vi "读取Description.vi"(8 "error in (no error)":errorcluster caption="错误输入（无错误）", 11 "Beverage输入":refnum<class "Beverage.lvclass">) -> (0 "error out":errorcluster caption="错误输出", 2 "Description":string="Unknown Description", 3 "Beverage输出":refnum<class "Beverage.lvclass">)   [LabVIEW 2016, in "Beverage.lvclass"]
uses:
  Beverage.lvclass
  Beverage.lvclass/Beverage.ctl
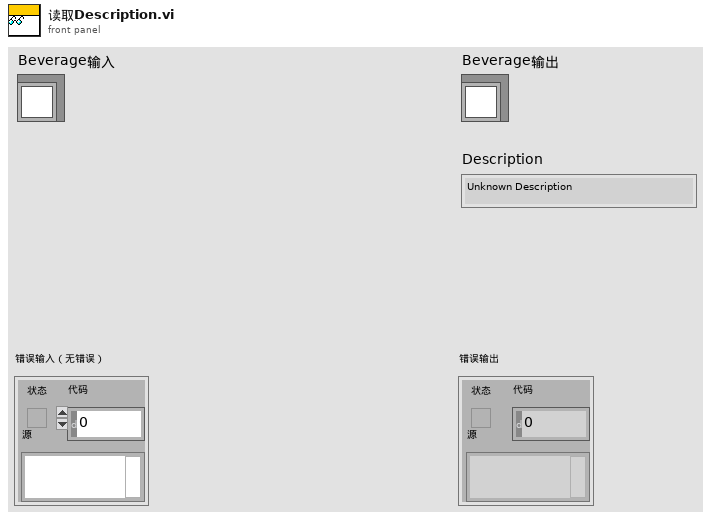
[diagram p1: front panel]
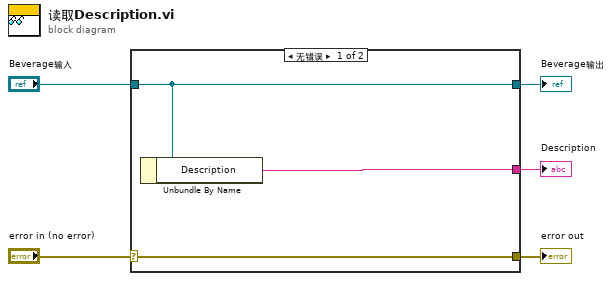
[diagram p0: block diagram]
diagram:
  n1 = case shown="无错误" "error in (no error)" {
    selector: "error in (no error)" -> [w8 w9]
    tunnel: [w8 w9] -> w4
    tunnel: [w7 w10] -> w2
    tunnel: "Beverage输入" -> [w7 w10]
    tunnel: [w6 _] -> w1
    frame No Error {
      n2 = Unbundle By Name(w7) -> ("Description"=w6:string)
    }
    frame Error {
    }
  }
  "error out" <- w4
  "Beverage输出" <- w2
  "Description" <- w1
